vi "main.vi"() -> ()   [LabVIEW 2013]
panel:
  in  "Parar":bool
  in  "Começar":bool
  out "Waveform Chart":dbl(graph)
  in  "stop":bool
  out "DDP":string
  out "Porta livre?":bool
  in  "baud rate (9600)":u32=9600
  in  "VISA Refnum in":refnum<visa-resource-name>="COM3"
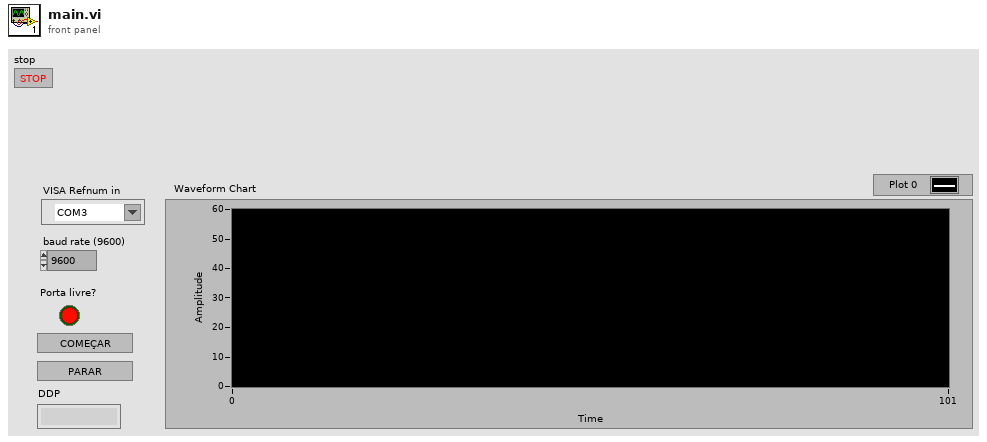
[diagram p1: front panel]
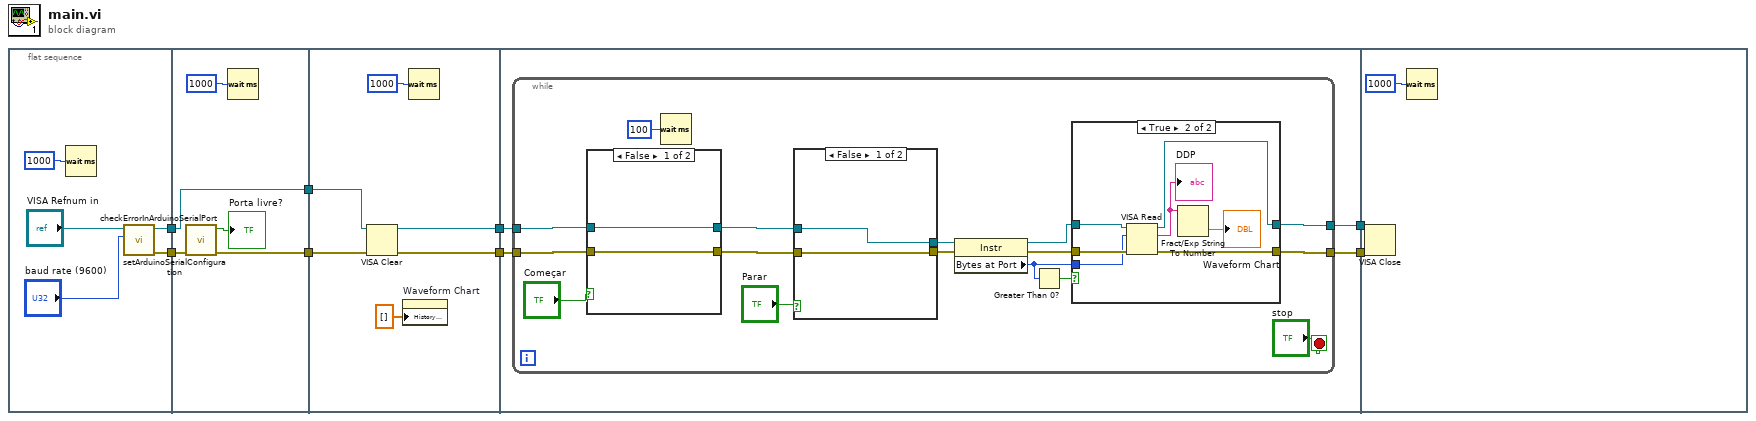
[diagram p0: block diagram]
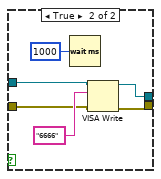
[diagram p2: hidden frame]
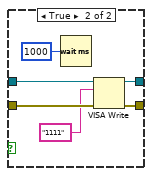
[diagram p3: hidden frame]
diagram:
  n1 = flat-sequence {
    tunnel: [w13] -> w6
    tunnel: [w12] -> w5
    tunnel: [w15] -> w8
    tunnel: [w18] -> w7
    tunnel: w6 -> [w18]
    tunnel: w5 -> [w16]
    tunnel: w8 -> [w24]
    tunnel: w7 -> [w23]
    tunnel: [w21] -> w2
    tunnel: [w20] -> w1
    tunnel: [w28] -> w4
    tunnel: [w27] -> w3
    tunnel: w1 -> [w25]
    tunnel: w2 -> [w26]
    tunnel: w4 -> [w71]
    tunnel: w3 -> [w70]
    frame #0 {
      n2 = Wait (ms)(milliseconds to wait=u32 1000) -> ()  [unwired: 1 out]
      n3 = call "setArduinoSerialConfiguration.vi"("baud rate (9600)"="baud rate (9600)", "VISA Refnum in"="VISA Refnum in") -> ("error out"=w12:errorcluster, "VISA Refnum out"=w13:refnum<visa-resource-name>)  [unwired: 8 in]
    }
    frame #1 {
      n4 = call "checkErrorInArduinoSerialPort.vi"("error in (no error)"=w16) -> ("error out"=w15:errorcluster, "Porta livre?"=→"Porta livre?":bool)  [unwired: 9 in]
      n5 = Wait (ms)(milliseconds to wait=u32 1000) -> ()  [unwired: 1 out]
    }
    frame #2 {
      n6 = VISA Clear(VISA resource name=w23, error in (no error)=w24) -> (VISA resource name out=w21:refnum<visa-resource-name>, error out=w20:errorcluster)
      n7 = property on="Waveform Chart" class="WFChart (strict)"("History Data"=dbl[] []) -> ()  [unwired: 2 in, 2 out]
      n8 = Wait (ms)(milliseconds to wait=u32 1000) -> ()  [unwired: 1 out]
    }
    frame #3 {
      n9 = while {
        tunnel: [w40] -> w28
        tunnel: [w42] -> w27
        tunnel: w26 -> [w37]
        tunnel: w25 -> [w36]
        stop <- "stop" stop-if-true
        n10 = case shown="False" "Começar" {
          tunnel: w37 -> [w54 w60]
          tunnel: w36 -> [w53 w58]
          tunnel: [w54 w59] -> w34
          tunnel: [w53 w57] -> w33
          frame False {
          }
          frame True {
            n11 = Wait (ms)(milliseconds to wait=u32 1000) -> ()  [unwired: 1 out]
            n12 = VISA Write(VISA resource name=w60, write buffer="1111", error in (no error)=w58) -> (VISA resource name out=w59:refnum<visa-resource-name>, error out=w57:errorcluster)  [unwired: 1 out]
          }
        }
        n13 = Wait (ms)(milliseconds to wait=u32 100) -> ()  [unwired: 1 out]
        n14 = case shown="False" "Parar" {
          tunnel: w34 -> [w45 w51]
          tunnel: w33 -> [w46 w49]
          tunnel: [w45 w50] -> w32
          tunnel: [w46 w48] -> w31
          frame False {
          }
          frame True {
            n15 = Wait (ms)(milliseconds to wait=u32 1000) -> ()  [unwired: 1 out]
            n16 = VISA Write(VISA resource name=w51, write buffer="6666", error in (no error)=w49) -> (VISA resource name out=w50:refnum<visa-resource-name>, error out=w48:errorcluster)  [unwired: 1 out]
          }
        }
        n17 = property class="Instr"(reference=w32, error in=w31) -> (reference out=w43:refnum<visa-resource-name>, error out=w41:errorcluster, "Bytes at Port"=w39:u32)
        n18 = Greater Than 0?(x=w39) -> (x > 0?=w44:bool)
        n19 = case shown="True" w44 {
          tunnel: w43 -> [w62 w69]
          tunnel: [w62 w68] -> w42
          tunnel: w41 -> [w61 w67]
          tunnel: [w61 w66] -> w40
          tunnel: w39 -> [_ w63]
          frame False {
          }
          frame True {
            n20 = VISA Read(VISA resource name=w69, byte count=w63, error in (no error)=w67) -> (VISA resource name out=w68:refnum<visa-resource-name>, read buffer=w65:string, error out=w66:errorcluster)  [unwired: 1 out]
            "DDP" <- w65
            n21 = Fract/Exp String To Number(string=w65) -> (number=→"Waveform Chart":dbl)  [unwired: 3 in, 1 out]
          }
        }
      }
    }
    frame #4 {
      n22 = VISA Close(VISA resource name=w70, error in (no error)=w71) -> ()  [unwired: 1 out]
      n23 = Wait (ms)(milliseconds to wait=u32 1000) -> ()  [unwired: 1 out]
    }
  }
